vi "LIN EX Ctrl Power Out.vi"(9 "VbatValue":u8, 10 "LINIndex":u8, 11 "DevHandle":i32) -> (3 "function return":i32)   [LabVIEW 2010, in "usb2lin_ex.lvlib"]
doc: "int WINAPI LIN_EX_CtrlPowerOut(int DevHandle,unsigned char LINIndex,unsigned char VbatValue);"
uses:
  usb2lin_ex.lvlib
  USB2XXX/trunk/USB2XXX/USB2XXX/vs2010/Release/USB2XXX.dll
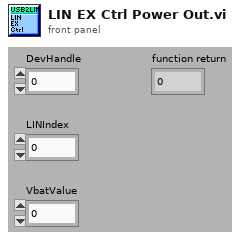
[diagram p1: front panel]
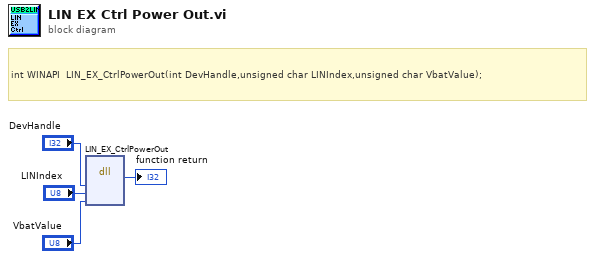
[diagram p0: block diagram]
diagram:
  # "int WINAPI  LIN_EX_CtrlPowerOut(int DevHandle,unsigned char LINIndex,unsigned char VbatValue);"
  n1 = dll-call lib="E:/Projects/USB2XXX/trunk/USB2XXX/USB2XXX/vs2010/Release/USB2XXX.*" fn="LIN_EX_CtrlPowerOut"("DevHandle"="DevHandle", "LINIndex"="LINIndex", "VbatValue"="VbatValue") -> (→"function return":i32)  [unwired: 6 in, 2 out]
